vi "Append Customized Table.vi"(0 "PDF Report IN":refnum<class "PDF Report Class.lvclass">, 3 "Row background color":T20={"color"=16777225, "at each"=0}, 5 "Table properties":T18={"Table position"=1, "SpacingBefore (points)"=0.0, "SpacingAfter (points)"=0.0} {"Table position" items=["LEFT", "CENTER", "RIGHT"]}, 7 "PDF Table":refnum<class "Pdfp Table Class.lvclass">, 9 "Caption":string, 11 "error in (no error)":errorcluster, 14 "Row  [ ]":T1) -> (4 "PDF Report OUT":refnum<class "PDF Report Class.lvclass">, 15 "error out":errorcluster)   [LabVIEW 2019, in "Exaprom PDF.lvlib"]
doc: "<B>ENGLISH</B>\nAppends a table to the PDF document.\n\n<B>FRANÇAIS</B>\nAjoute un tableau au document PDF.\n\nVersion 2.0\nDeveloped by Jean-Marc Simard\nCopyright © 2012, Exaprom Inc.\nAll rights reserved.\nLicense: BSD\n\nWith iTextSharp 4.1.6 (http://itextsharp.sourceforge.net)\nunder Mozilla Public License Version 1.1\n(http://www.mozilla.org/MPL/MPL-1.1.html)"
uses:
  LV Class/PDF Report Class/PDF Report Class.lvclass
  Controls/Table Controls/Row Back Ground color Datas.ctl
  Controls/Table Controls/Table properties.ctl
  Controls/Table Controls/Table position.ctl
  LV Class/Pdfp Table Class/Pdfp Table Class.lvclass
  Controls/Table Controls/Table Appearance and Font Row [ ].ctl
  Controls/Table Controls/One Row Appearance.ctl
  Controls/Table Controls/Row from to.ctl
  Controls/Table Controls/Cell, Alignment, LS and Font - hide Vmerge.ctl
  Controls/Table Controls/Cell Type, Alignment and LS.ctl
  Controls/Table Controls/Cell Alignment 20px.ctl
  Controls/Table Controls/Text vertical arrangement.ctl
  Controls/Text Controls/Line spacing.ctl
  Controls/Table Controls/Cell Appearance.ctl
  Controls/Table Controls/Cell Border 20 px.ctl
  Controls/Table Controls/Merge Horizontal.ctl
  Controls/Table Controls/Merge Vertical.ctl
  Controls/Font Controls/Font complete cluster.ctl
  Controls/Font Controls/Font size.ctl
  Controls/Font Controls/Font color.ctl
  Controls/Font Controls/Type and encoding.ctl
  Controls/Text Controls/Unicode/Type and run direction.ctl
  Exaprom PDF.lvlib
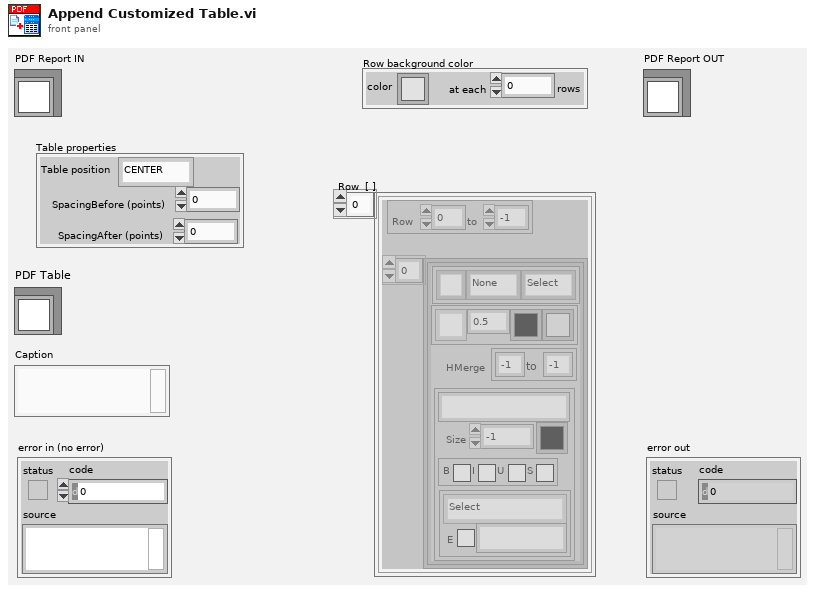
[diagram p1: front panel]
types:
  T1 = typedef "Exaprom PDF.lvlib/Table Appearance and Font Row [ ].ctl" = T2[]
  T2 = typedef "Exaprom PDF.lvlib/One Row Appearance.ctl" = cluster{"Row":T3, "Cell [ ]":T4[]}
  T3 = typedef "Exaprom PDF.lvlib/Row from to.ctl" = cluster{"From #":i16, "to #":i16}
  T4 = typedef "Exaprom PDF.lvlib/Cell, Alignment, LS and Font - hide Vmerge.ctl" = cluster{"Text":T5, "Cell Appearance":T9, "HMerge":T11, "VMerge":T12, "Font":T13}
  T5 = typedef "Exaprom PDF.lvlib/Cell Type, Alignment and LS.ctl" = cluster{"Cell Alignment":T6, "Text rotation":T7, "Line spacing":T8}
  T6 = typedef "Exaprom PDF.lvlib/Cell Alignment 20px.ctl" = u16
  T7 = typedef "Exaprom PDF.lvlib/Text vertical arrangement.ctl" = enum16{"None", "Clockwise", "Counterclockwise"}
  T8 = typedef "Exaprom PDF.lvlib/Line spacing.ctl" = enum16{"Select", "1.0", "1.5", "2.0"}
  T9 = typedef "Exaprom PDF.lvlib/Cell Appearance.ctl" = cluster{"Border":T10, "Thickness":sgl, "Color":u32, "BG":u32}
  T10 = typedef "Exaprom PDF.lvlib/Cell Border 20 px.ctl" = u16
  T11 = typedef "Exaprom PDF.lvlib/Merge Horizontal.ctl" = cluster{"From":i8, "to":i8}
  T12 = typedef "Exaprom PDF.lvlib/Merge Vertical.ctl" = cluster{"From":i8, "to":i8}
  T13 = typedef "Exaprom PDF.lvlib/Font complete cluster.ctl" = cluster{"Name":string, "Size":T14, "Color":T15, "Style":cluster{"Bold":bool, "Italic":bool, "Underline":bool, "Strikeout":bool}, "Type":T16}
  T14 = typedef "Exaprom PDF.lvlib/Font size.ctl" = sgl
  T15 = typedef "Exaprom PDF.lvlib/Font color.ctl" = u32
  T16 = typedef "Exaprom PDF.lvlib/Type and encoding.ctl" = cluster{"Type&direction":T17, "Embedded":bool, "Encoding":string}
  T17 = typedef "Exaprom PDF.lvlib/Type and run direction.ctl" = enum16{"Select", "ASCII", "UTF-16", "UTF-16 (default)", "UTF-16 (LTR)", "UTF-16 (RTL)"}
  T18 = typedef "Exaprom PDF.lvlib/Table properties.ctl" = cluster{"Table position":T19, "SpacingBefore (points)":sgl, "SpacingAfter (points)":sgl}
  T19 = typedef "Exaprom PDF.lvlib/Table position.ctl" = i32
  T20 = typedef "Exaprom PDF.lvlib/Row Back Ground color Datas.ctl" = cluster{"color":u32, "at each":i16}
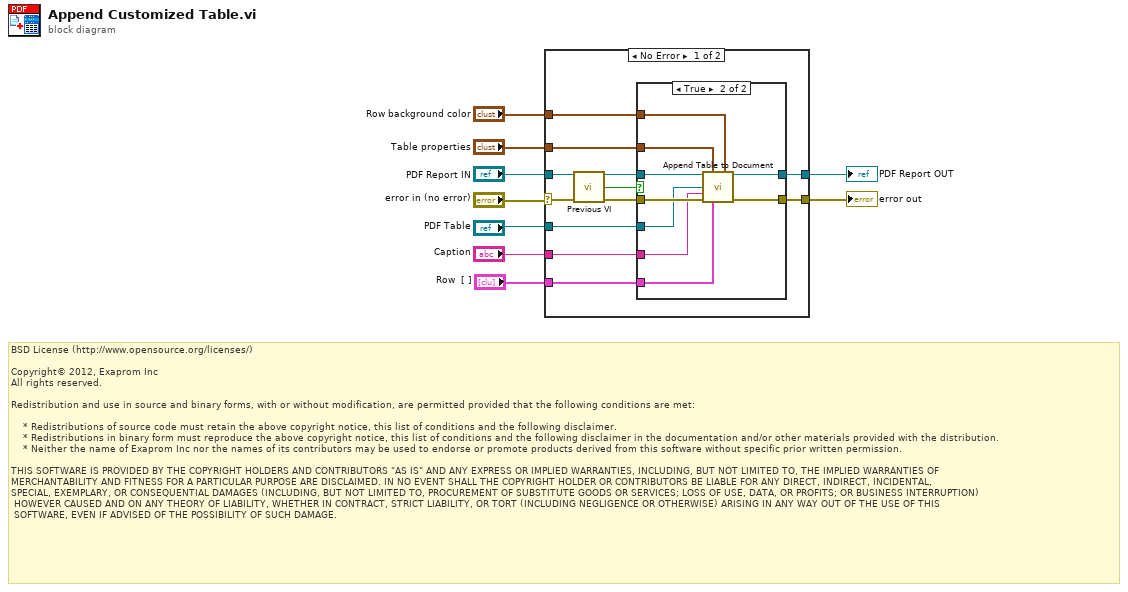
[diagram p0: block diagram]
diagram:
  # "BSD License (http://www.opensource.org/licenses/)\n\nCopyright© 2012, Exaprom Inc\nAll rights reserved.\n\nRedistribution and use in source and binary forms, with or without modification, are permitted provided that the following conditions are met:\n\n    * Redistributions of source code must retain the above copyright notice, this list of conditions and the following disclaimer.\n    * Redistributions in binary form must reproduce the above copyright notice, this list of conditions and the following disclaimer in the documentation and/or other materials provided with the distribution.\n    * Neither the name of Exaprom Inc nor the names of its contributors may be used to endorse or promote products derived from this software without specific prior written permission.\n\nTHIS SOFTWARE IS PROVIDED BY THE COPYRIGHT HOLDERS AND CONTRIBUTORS \"AS IS\" AND ANY EXPRESS OR IMPLIED WARRANTIES, INCLUDING, BUT NOT LIMITED TO, THE IMPLIED WARRANTIES OF \nMERCHANTABILITY AND FITNESS FOR A PARTICULAR PURPOSE ARE DISCLAIMED. IN NO EVENT SHALL THE COPYRIGHT HOLDER OR CONTRIBUTORS BE LIABLE FOR ANY DIRECT, INDIRECT, INCIDENTAL,\nSPECIAL, EXEMPLARY, OR CONSEQUENTIAL DAMAGES (INCLUDING, BUT NOT LIMITED TO, PROCUREMENT OF SUBSTITUTE GOODS OR SERVICES; LOSS OF USE, DATA, OR PROFITS; OR BUSINESS INTERRUPTION)\n HOWEVER CAUSED AND ON ANY THEORY OF LIABILITY, WHETHER IN CONTRACT, STRICT LIABILITY, OR TORT (INCLUDING NEGLIGENCE OR OTHERWISE) ARISING IN ANY WAY OUT OF THE USE OF THIS\n SOFTWARE, EVEN IF ADVISED OF THE POSSIBILITY OF SUCH DAMAGE."
  n1 = case shown="No Error" "error in (no error)" {
    selector: "error in (no error)" -> [w16 w33]
    tunnel: "Table properties" -> [w21 _]
    tunnel: "PDF Report IN" -> [w14 w34]
    tunnel: "Caption" -> [w20 _]
    tunnel: "Row background color" -> [w19 _]
    tunnel: [w18 w34] -> w4
    tunnel: [w17 w33] -> w3
    tunnel: "PDF Table" -> [w12 _]
    tunnel: "Row  [ ]" -> [w11 _]
    frame No Error {
      n2 = call "Previous VI.vi"("PDF Report IN"=w14, "error in (no error)"=w16) -> ("PDF Report OUT"=w13:refnum<class "PDF Report Class.lvclass">, "Execute Actual VI"=w10:bool, "error out"=w15:errorcluster)  [unwired: 11 out]
      n3 = case shown="True" w10 {
        tunnel: w21 -> [_ w27]
        tunnel: w20 -> [_ w25]
        tunnel: w19 -> [_ w28]
        tunnel: [w23 w30] -> w18
        tunnel: [w22 w31] -> w17
        tunnel: w15 -> [w22 w32]
        tunnel: w13 -> [w23 w29]
        tunnel: w12 -> [_ w26]
        tunnel: w11 -> [_ w24]
        frame False {
        }
        frame True {
          n4 = call "Append Table to Document.vi"("PDF Report IN"=w29, "Table properties"=w27, "Row background color"=w28, "PDF Table"=w26, "Caption"=w25, "error in (no error)"=w32, "Row  [ ]"=w24) -> ("PDF Report OUT"=w30:refnum<class "PDF Report Class.lvclass">, "error out"=w31:errorcluster)  [unwired: 7 in]
        }
      }
    }
    frame Error {
    }
  }
  "error out" <- w3
  "PDF Report OUT" <- w4
